vi "SubPanel_DataCollection_Rev11_v10.vi"(0 "DCPowerInformationClusterArray_Input":T7(array[cluster]), 1 "VISAPowerInfoInputArray":T6(array[cluster]), 2 "Run Data SubPanel Input":T5, 3 "RF Block Parameters":T4, 4 "Oscilloscope Info Array":T3(array[cluster]) {"vertical coupling" items=["AC", "DC", "Ground"]}, 6 "New Run?":bool, 7 "error in":errorcluster) -> (20 "DCPowerInformationClusterArray_Output":T7(array[cluster]), 21 "VISAPowerInfoInputOutput":T6(array[cluster]), 22 "Run Data SubPanel Output":T5, 23 "RF Block Parameters Output":T4, 24 "Oscilloscope Info Array Output":T3(array[cluster]) {"vertical coupling" items=["AC", "DC", "Ground"]}, 25 "Reinitialize?":bool, 26 "Data Was Collected?":bool, 27 "error out":errorcluster)   [LabVIEW 2019]
uses:
  Controls/DataBlockControl.ctl
  Controls/QueueDataControl_V3.ctl
  <vilib>/Utility/file.llb/Write Delimited Spreadsheet (string).vi
  Controls/RFBlockControl.ctl
  <instrlib>/niScope/Controls/niScope vertical coupling.ctl
panel:
  out "Current Measurements Live Total":T1(graph)
  out "Voltage Measurements Live Total":T1(graph)
  out "Voltage Measurements Live":T1(graph)
  out "Current Measurements Live":T1(graph)
  out "DCPowerInfoArray":string[][](array[string])
  out "Array":string[][][](array[string])
  out "Current Measurements":cluster{dbl[], dbl[]}[](graph)
  out "Voltage Measurements":cluster{dbl[], dbl[]}[](graph)
  out "Exiting":bool
  out "Full Run Information":string
  out "Ready For Next Run?":bool
  in  "Next Run":bool
  out "Recording Data":bool
  out "Current 2":waveform(dbl)[](graph)
  out "Voltage 2":waveform(dbl)[](graph)
  in  "Record Data Toggle":bool
  out "error of collection":errorcluster
  in  "force exit SubVI":bool
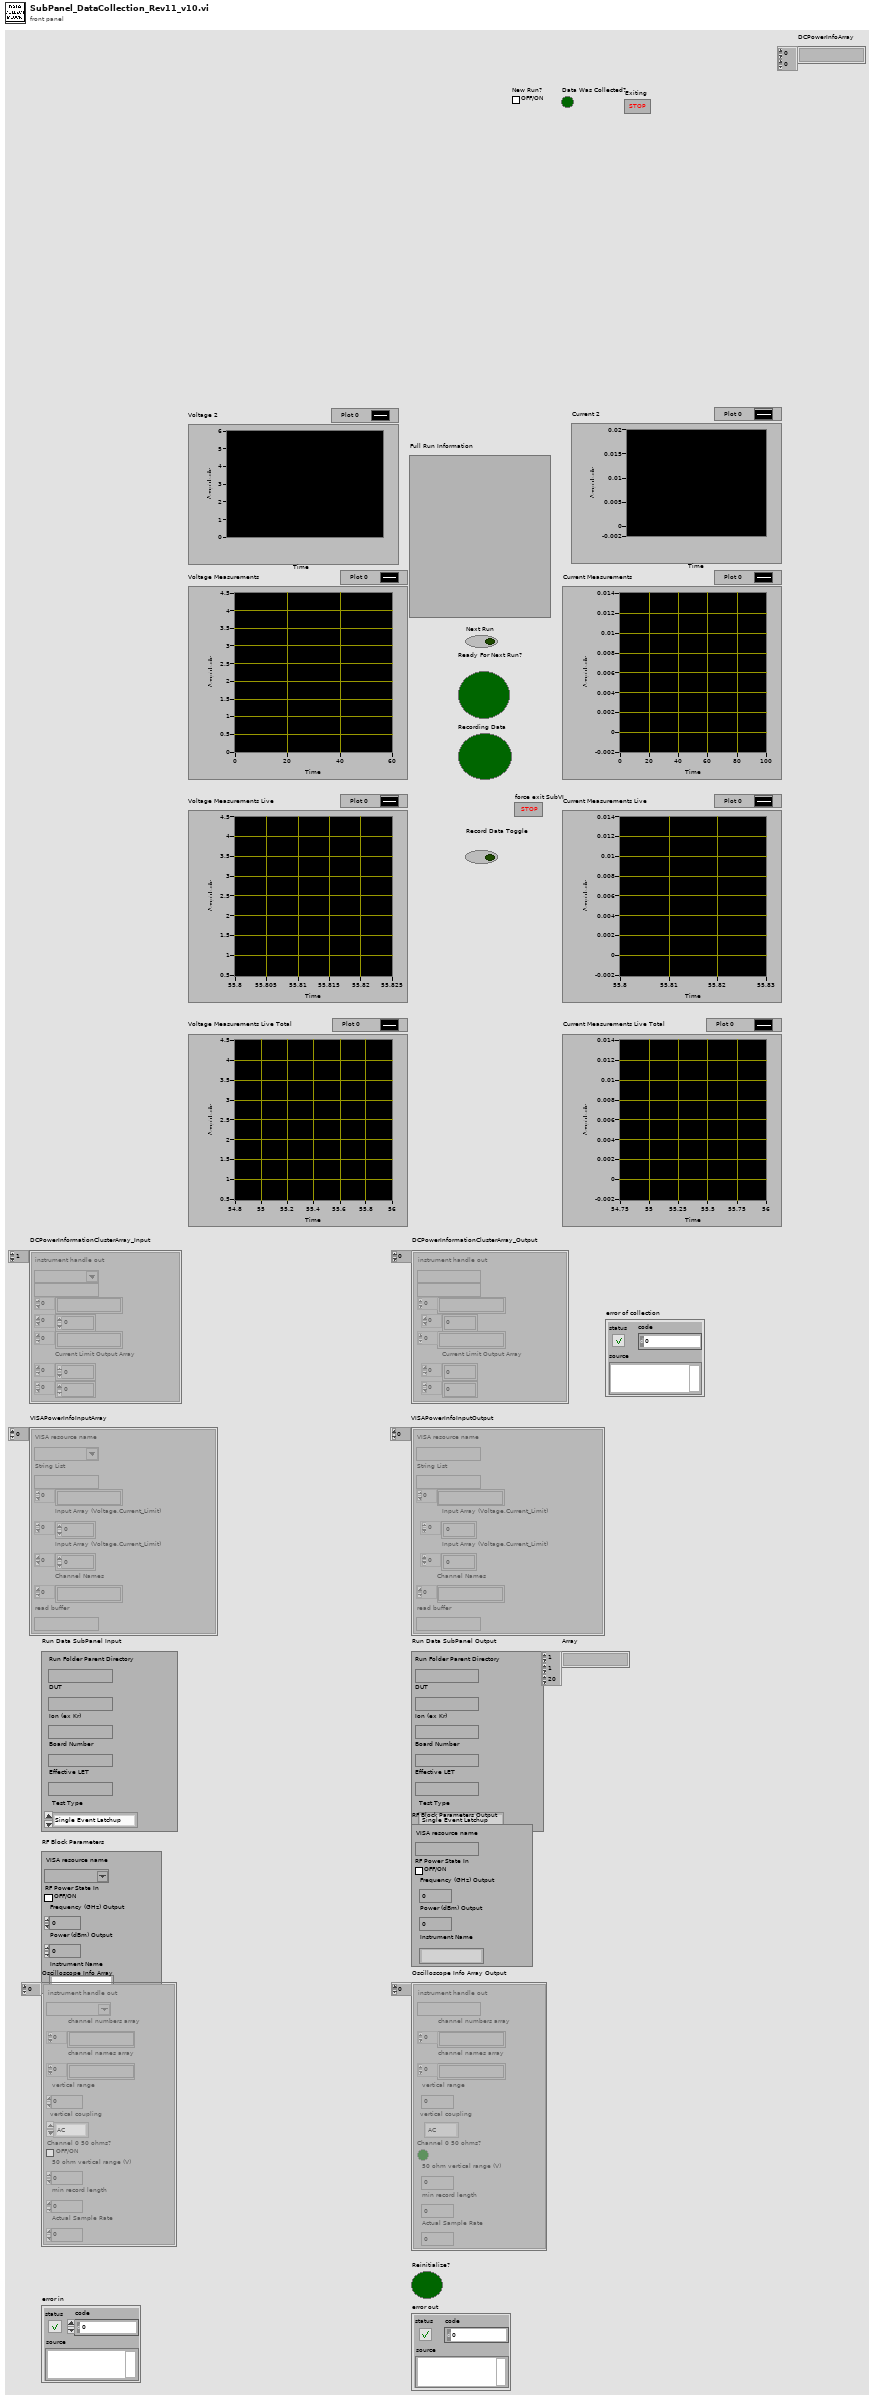
[diagram p1: front panel]
types:
  T1 = cluster{"Array of fetched data":dbl[], "Array of fetched data":dbl[]}[]
  T2 = typedef "niScope vertical coupling.ctl" = i32
  T3 = cluster{"instrument handle out":refnum<k15>, "channel numbers array":string[], "channel names array":string[], "vertical range":dbl, "vertical coupling":T2, "Channel 0 50 ohms?":bool, "50 ohm vertical range (V)":dbl, "min record length":i32, "Actual Sample Rate":dbl}[]
  T4 = typedef "RFBlockControl.ctl" = cluster{"VISA resource name":refnum<visa-resource-name>, "RF Power State In":bool, "Frequency (GHz) Output":dbl, "Power (dBm) Output":dbl, "Instrument Name":string}
  T5 = typedef "DataBlockControl.ctl" = cluster{"Run Folder Parent Directory":path, "DUT":string, "Ion (ex Kr)":string, "Board Number":string, "Effective LET":string, "Test Type":enum16{"Single Event Latchup", "Single Event Transient", "Single Event Upset"}}
  T6 = cluster{"VISA resource name":refnum<visa-resource-name>, "String List":string, string[], "Input Array (Voltage,Current_Limit)":dbl[], "Input Array (Voltage,Current_Limit)":dbl[], "Channel Names":string[], "read buffer":string}[]
  T7 = cluster{"instrument handle out":refnum<k15>, string, string[], dbl[], string[], "Current Limit Output Array":dbl[], dbl[]}[]
  T8 = typedef "QueueDataControl_V3.ctl" = cluster{"Array of fetched data":dbl[][][], "Channel Names Array":string[], "Voltage Waveform Array":waveform(dbl)[], "Current Waveform Array":waveform(dbl)[], "Resetting Time":timestamp}
  T9 = cluster{"IVI Refnum out":refnum<k15>, string, "voltage level channel 23":dbl, "Channel Name 23":string, "Current Limit":dbl, "Measure Record dt":dbl, string}[]
  T10 = cluster{"created path":path, "DCPowerInformation_byChannel":cluster{"IVI Refnum out":refnum<k15>, string, "voltage level channel 23":dbl, "Channel Name 23":string, "Current Limit":dbl, "Measure Record dt":dbl, string}[], string[]}
  T11 = cluster{"Array of fetched data":dbl[][], string, i32[]}
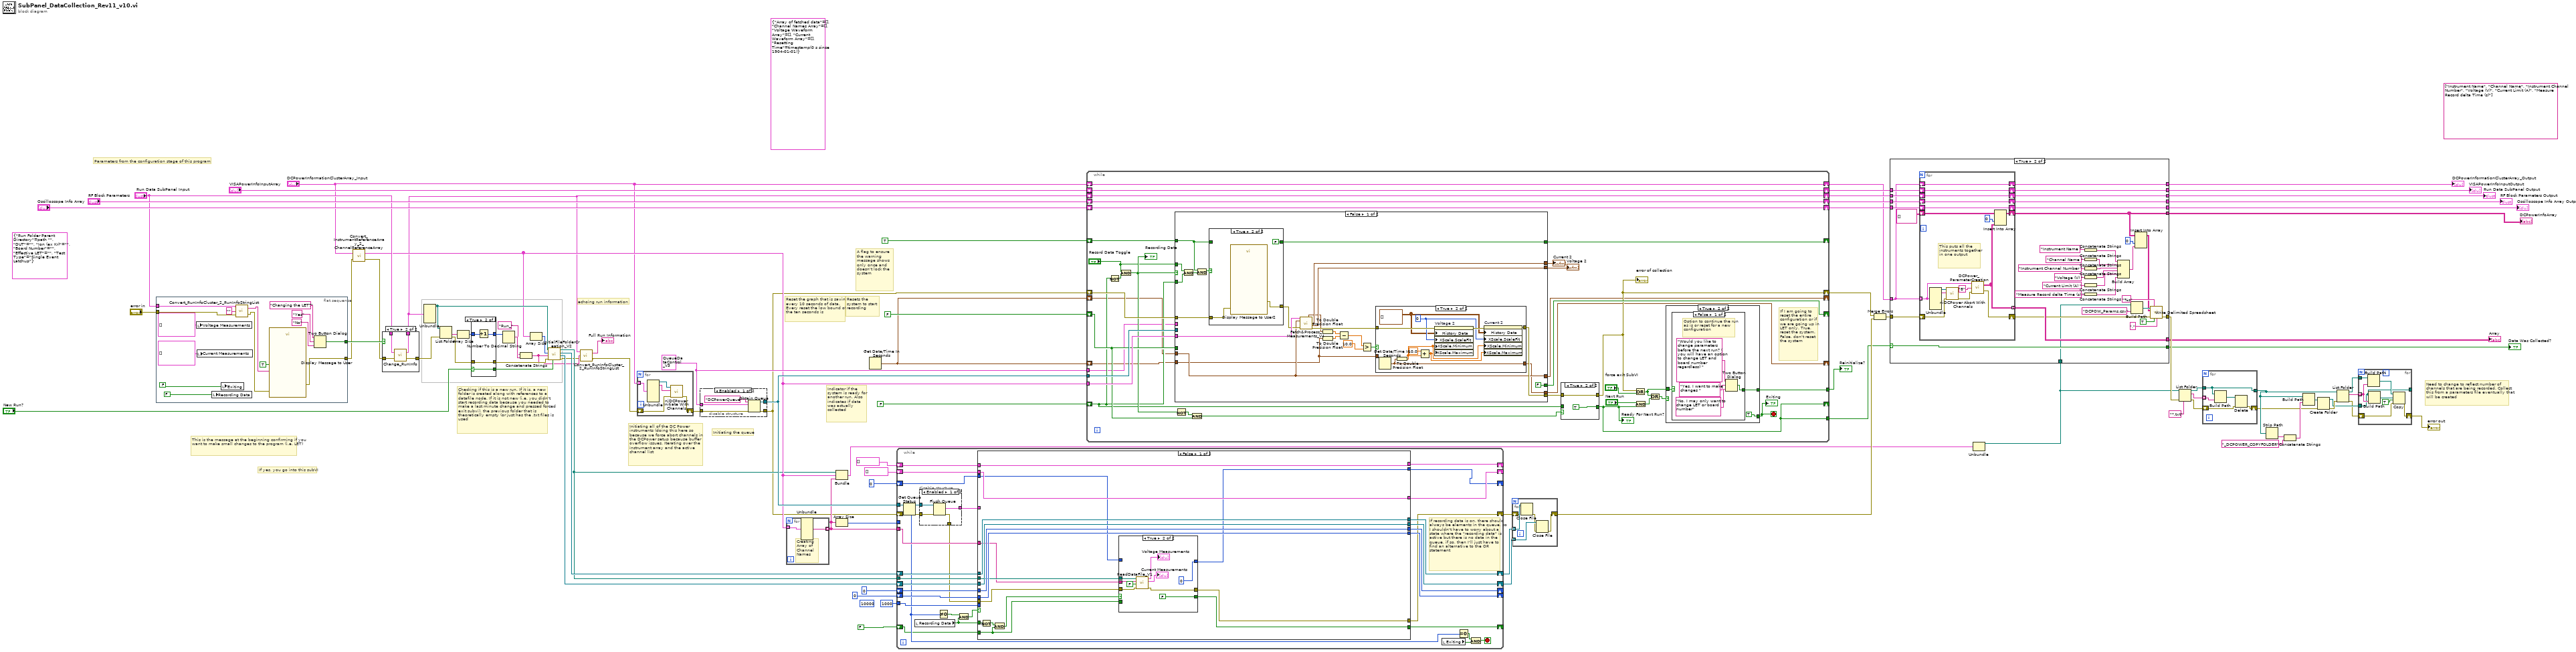
[diagram p0: block diagram]
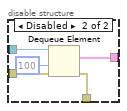
[diagram p2: hidden frame]
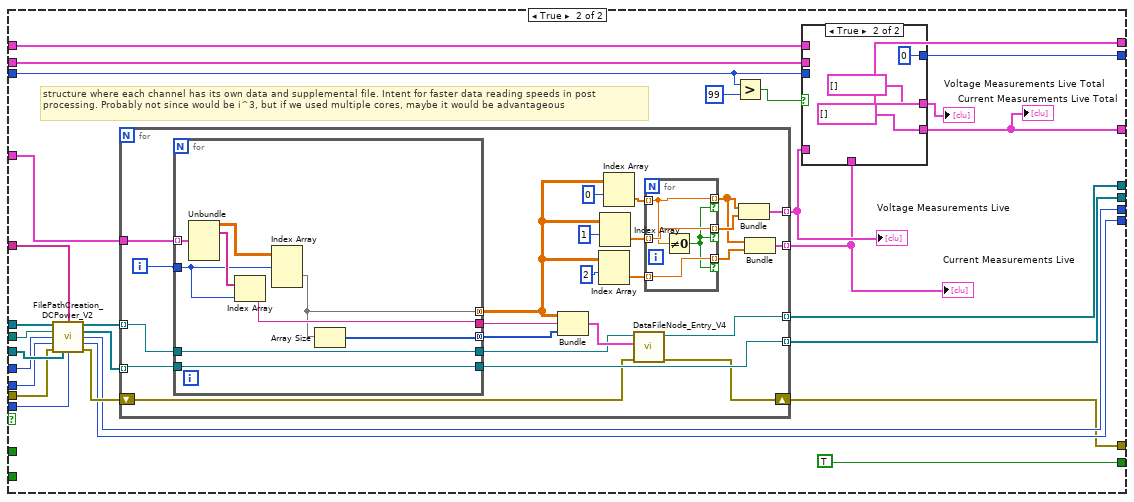
[diagram p4: hidden frame]
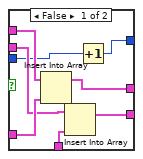
[diagram p5: hidden frame]
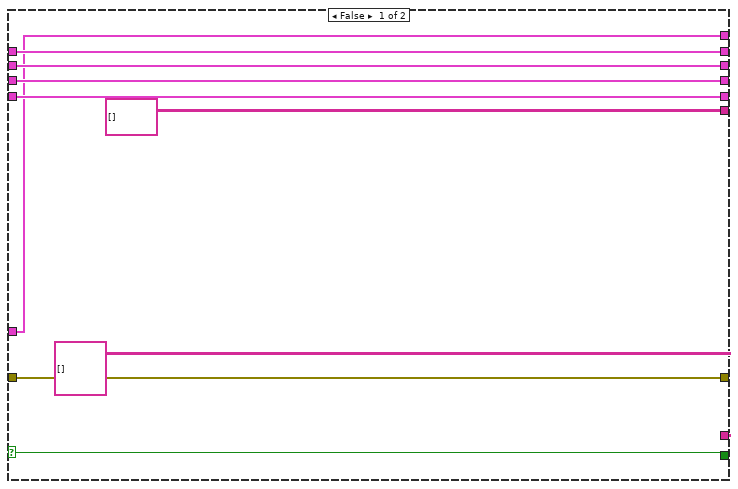
[diagram p6: hidden frame]
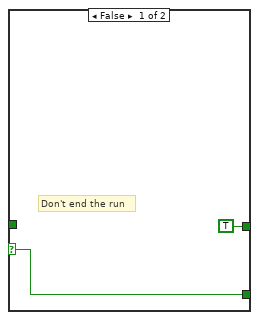
[diagram p10: hidden frame]
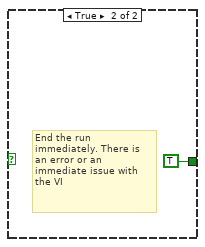
[diagram p11: hidden frame]
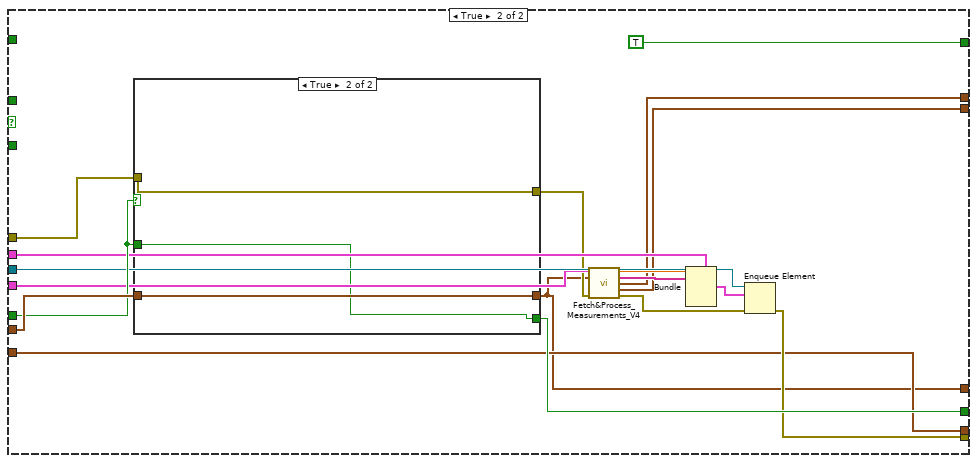
[diagram p15: hidden frame]
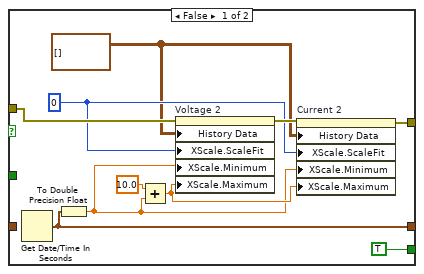
[diagram p16: hidden frame]
diagram:
  (unwired) string[] ["Instrument Name", "Channel Name", "Instrument Channel Number", "Voltage (V)", "Current Limit (A)", "Measure Record delta Time (s)"] ("new element/subarray")
  w57 = T8 {"Array of fetched data"=[], "Channel Names Array"=[], "Voltage Waveform Array"=[], "Current Waveform Array"=[], "Resetting Time"=timestamp(0 s since 1904-01-01)} ("DCPower Queue Data Double Array Format")
  (unwired) T8 {"Array of fetched data"=[], "Channel Names Array"=[], "Voltage Waveform Array"=[], "Current Waveform Array"=[], "Resetting Time"=timestamp(0 s since 1904-01-01)} ("DCPower Double Array Queue")
  (unwired) 10000 ("binary file indexor in")
  (unwired) T5 {"Run Folder Parent Directory"=path "", "DUT"="", "Ion (ex Kr)"="", "Board Number"="", "Effective LET"="", "Test Type"=enum."Single Event Latchup"} ("Run Data Configuration")
  # "Initiating the queue"
  # "echoing run information"
  # "Checking if this is a new run. If it is, a new folder is created along with references to a datafile node. If it is not new (i.e. you didn't start recording data because you needed to make a last minute change and pressed forced exit subvi), the previous folder that is theoretically empty (or just has the .txt files is used"
  # "If yes, you go into this subVI"
  # "This is the message at the beginning confirming if you want to make small changes to the program (i.e. LET)"
  # "Parameters from the configuration stage of this program"
  # "Reset the graph that is saving every 10 seconds of data. Every reset the low bound of the ten seconds is"
  # "Need to change to reflect number of channels that are being recorded. Collect this from a parameters file eventually that will be created"
  # "Indicator if the system is ready for another run. Also indicates if data was actually collected"
  # "Resets the system to start recording"
  # "A flag to ensure the warning message shows only once and doesn't lock the system"
  # "Initiating all of the DC Power instruments (doing this here so because we force abort channels in the DCPower setup because buffer overflow issues. Iterating over the instrument array and the active channel list"
  n1 = flat-sequence {
    tunnel: [w98] -> w73
    tunnel: "error in" -> [w90]
    tunnel: [w102] -> w78
    tunnel: "Run Data SubPanel Input" -> [w89]
    frame #0 {
      n2 = local write "Voltage Measurements"(cluster{dbl[], dbl[]}[] [] ("Voltage Measurements")) -> ()
      n3 = local write "Current Measurements"(cluster{dbl[], dbl[]}[] [] ("Current Measurements")) -> ()
      n4 = local write "Recording Data"(FALSE ("Recording Data")) -> ()
      n5 = local write "Exiting"(FALSE ("Forced Exit")) -> ()
      n6 = call "Convert_RunInfoCluster_2_RunInfoStringList.vi"("error in"=w90, "Run Number"="", "Run Data SubPanel Input"=w89) -> ("error output"=w91:errorcluster, "Run Data Output"=w92:string)
      n7 = call "Display Message to User"("error in (no error)"=w91, "Enable"=TRUE, "Message"=w92) -> ("error out"=w98:errorcluster)  [unwired: 7 in, 1 out]
      n8 = Two Button Dialog(message="Changing the LET?", 1:"No" ("F button name (\"Cancel\")"), 2:"Yes" ("T button name (\"OK\")")) -> (T button?=w102:bool)
    }
  }
  n9 = call "Convert_InstrumentReferenceArray_2_ChannelReferenceArray.vi"("error in (no error)"=w73, "DCPowerInformationClusterArray_Input"="DCPowerInformationClusterArray_Input") -> ("error out"=w72:errorcluster, "DCPowerInformation_byChannel"=w30:T9)
  n10 = case shown="True" w78 {
    tunnel: "Run Data SubPanel Input" -> [w104 w108]
    tunnel: [w104 w107] -> w7
    tunnel: [w103 w106] -> w74
    tunnel: w72 -> [w103 w105]
    frame False {
    }
    frame True {
      n11 = call "Change_RunInfo.vi"("error in (no error)"=w105, "Run Data SubPanel in"=w108) -> ("error out"=w106:errorcluster, "Run Data SubPanel out"=w107:T5)
    }
  }
  n12 = Unbundle(w7) -> ("Run Folder Parent Directory"=w75:path)  [unwired: 5 out]
  n13 = List Folder(path=w75, error in=w74) -> (folder names=w76:string[], error out=w60:errorcluster)  [unwired: 2 in, 2 out]
  n14 = Array Size(array=w76) -> (size(s)=w63:i32)
  n15 = case shown="True" "New Run?" {
    selector: "New Run?" -> [w110 w113]
    tunnel: [w111 w115] -> w64
    tunnel: w63 -> [w111 w114]
    tunnel: [w110 w113] -> w62
    tunnel: [w109 w112] -> w61
    tunnel: w60 -> [w109 w112]
    frame False {
    }
    frame True {
      n16 = Increment(x=w114) -> (x+1=w115:i32)
    }
  }
  n17 = Number To Decimal String(number=w64) -> (decimal integer string=w67:string)  [unwired: 1 in]
  n18 = Concatenate Strings("Run_", w67) -> (w6:string)
  n19 = Array Size(array=w30) -> (size(s)=w59:i32)
  n20 = call "InitialFileFolderCreation_V2.vi"("New Run?"=w62, "error in (no error)"=w61, "Run Number"=w6, "DCPowerArrayClusterSize"=w59, "base path"=w75) -> ("error out"=w5:errorcluster, "SupplementalDataFileReferenceObjectArray"=w70:refnum<file>[], "DataFileReferenceObjectArray"=w71:refnum<file>[], "created path"=w14:path)  [unwired: 3 in]
  n21 = call "Convert_RunInfoCluster_2_RunInfoStringList.vi"("error in"=w5, "Run Number"=w6, "Run Data SubPanel Input"=w7) -> ("error output"=w4:errorcluster, "Run Data Output"=→"Full Run Information":string)
  n22 = for {
    shift-right: [w116] -> w12
    shift-left: w4 -> [w118]
    tunnel: "DCPowerInformationClusterArray_Input" -> [w120] mode=indexing
    n23 = Unbundle(w120) -> ("instrument handle out"=w117:refnum<k15>, w119:string)  [unwired: 5 out]
    n24 = call <instrlib>:"niDCPower Initiate With Channels.vi"("error in (no error)"=w118, "channel name"=w119, "instrument handle"=w117) -> ("error out"=w116:errorcluster)  [unwired: 7 in, 1 out]
  }
  n25 = disable-structure shown="Enabled" {
    disable-tunnel: w12 -> [w124 w126]
    disable-tunnel: [w123 w126] -> w9
    disable-tunnel: [w122 _] -> w83
    disable-tunnel: w57 -> [w121 _]
    frame Enabled {
      n26 = Obtain Queue(name (unnamed)="DCPowerQueue", element data type=w121, error in (no error)=w124) -> (queue out=w122:refnum<queue>, error out=w123:errorcluster)  [unwired: 2 in, 1 out]
    }
    frame Disabled {
    }
  }
  n27 = for {
    tunnel: w30 -> [w128] mode=indexing
    tunnel: [w127] -> w31 mode=indexing
    # "Creating Array of Channel Names"
    n28 = Unbundle(w128) -> ("Channel Name 23"=w127:string)  [unwired: 6 out]
  }
  n29 = Bundle("created path"=w14, "DCPowerInformation_byChannel"=w30, w31) -> (w29:T10)  [unwired: 1 in]
  n30 = Array Size(array=w31) -> (size(s)=w52:i32)
  n31 = Get Date/Time In Seconds() -> (seconds since 1Jan1904=w10:timestamp)
  n32 = while {
    tunnel: w83 -> [w161]
    shift-right: [w148] -> w54
    shift-left: w9 -> [w160]
    tunnel: w14 -> [w157]
    shift-right: [w150] -> w56
    shift-left: w71 -> [w158]
    shift-right: [w149] -> w55
    shift-left: w70 -> [w156]
    shift-right: [w152] -> _
    shift-left: 0 ("binary file indexor in") -> [w155]
    shift-right: [w151] -> _
    shift-left: 0 ("binary file indexor in") -> [w154]
    tunnel: 1000 ("binary file indexor in") -> [w153]
    tunnel: w31 -> [w159]
    tunnel: w52 -> [_]
    shift-right: [w137] -> _
    shift-left: FALSE -> [w136]
    shift-right: [w133] -> _
    shift-left: T1 [] ("array") -> [w134]
    shift-right: [w131] -> _
    shift-left: T1 [] ("array") -> [w132]
    shift-right: [w129] -> _
    shift-left: 0 -> [w130]
    stop <- w145 stop-if-true
    # "If recording data is on, there should always be elements in the queue, so I shouldn't have to worry about a state where the \"recording data\" is active but there is no data in the queue, if so, then I'll just have to find an alternative to the OR statement"
    n33 = Get Queue Status(queue=w161, error in (no error)=w160) -> (queue out=w142:refnum<queue>, error out=w143:errorcluster, # elements in queue=w138:i32)  [unwired: 1 in, 5 out]
    n34 = local read "Recording Data"() -> (w135:bool)
    n35 = disable-structure shown="Enabled" {
      disable-tunnel: [w165 w167] -> w144
      disable-tunnel: w143 -> [w164 w169]
      disable-tunnel: w142 -> [w163 w170]
      disable-tunnel: [w162 w166] -> w141
      frame Enabled {
        n36 = Flush Queue(queue=w163, error in (no error)=w164) -> (remaining elements=w162:T8[], error out=w165:errorcluster)  [unwired: 1 out]
      }
      frame Disabled {
        n37 = Dequeue Element(queue=w170, timeout in ms (-1)=100, error in (no error)=w169) -> (element=w166:T8, error out=w167:errorcluster)  [unwired: 2 out]
      }
    }
    n38 = Not Equal To 0?(x=w138) -> (x != 0?=w140:bool)
    n39 = And(x=w140, y=w135) -> (x .and. y?=w139:bool)
    n40 = case shown="False" w139 {
      tunnel: w141 -> [_ w227]
      tunnel: w144 -> [w178 w221]
      tunnel: w159 -> [w179 w213]
      tunnel: w158 -> [w186 w226]
      tunnel: w157 -> [w180 w225]
      tunnel: w156 -> [w187 w224]
      tunnel: w155 -> [w185 w223]
      tunnel: w154 -> [w184 w212]
      tunnel: w153 -> [_ w211]
      tunnel: [w185 w220] -> w152
      tunnel: [w184 w219] -> w151
      tunnel: [w186 w216] -> w150
      tunnel: [w187 w215] -> w149
      tunnel: [w177 w214] -> w148
      tunnel: [w176 TRUE] -> w137
      tunnel: w136 -> [w175 _]
      tunnel: w135 -> [w183 _]
      tunnel: w134 -> [w174 w207]
      tunnel: [w174 w206] -> w133
      tunnel: w132 -> [w173 w205]
      tunnel: [w173 w204] -> w131
      tunnel: w130 -> [w172 w201]
      tunnel: [w171 w200] -> w129
      frame False {
        n41 = Not(x=w183) -> (.not. x?=w182:bool)
        n42 = And(x=w182, y=w175) -> (x .and. y?=w181:bool)
        n43 = case shown="True" w181 {
          tunnel: w180 -> [_ w199]
          tunnel: w179 -> [_ w198]
          tunnel: w178 -> [w190 w196]
          tunnel: [w190 w195] -> w177
          tunnel: [w189 FALSE] -> w176
          tunnel: w175 -> [w189 _]
          tunnel: w172 -> [w188 _]
          tunnel: [w188 0] -> w171
          frame False {
          }
          frame True {
            n44 = call "ReadDataFile_V1.vi"("error in (no error)"=w196, "Create CSV files?"=FALSE, "Channel Names Array"=w198, "DataFolder Path"=w199) -> ("error out"=w195:errorcluster, "Current Measurements"=→"Current Measurements":cluster{dbl[], dbl[]}[], "Voltage Measurements"=→"Voltage Measurements":cluster{dbl[], dbl[]}[])  [unwired: 5 in]
          }
        }
      }
      frame True {
        # "structure where each channel has its own data and supplemental file. Intent for faster data reading speeds in post processing. Probably not since would be i^3, but if we used multiple cores, maybe it would be advantageous"
        n45 = call "FilePathCreation_DCPower_V2.vi"("binary file input reference array 1"=w226, "Channel Name Input array"=w213, "data output directory folder"=w225, "binary file indexor in"=w223, "Reset counter in"=w212, "error in (no error)"=w221, "binary file input reference array 2"=w224, "reset threshold"=w211) -> ("binary file output reference array"=w218:refnum<file>[], "binary file output reference array 2"=w217:refnum<file>[], "binary file indexor out"=w220:i32, "reset counter out"=w219:i32, "error out"=w222:errorcluster)  [unwired: 3 in]
        n46 = for {
          shift-right: [w252] -> w214
          shift-left: w222 -> [w253]
          tunnel: w227 -> [w262]
          tunnel: w217 -> [w259] mode=indexing
          tunnel: w218 -> [w258] mode=indexing
          tunnel: [w257] -> w215 mode=indexing
          tunnel: [w251] -> w216 mode=indexing
          tunnel: [w246] -> w209 mode=indexing
          tunnel: [w245] -> w208 mode=indexing
          i -> [w256]
          n47 = for {
            tunnel: w262 -> [w275] mode=indexing
            tunnel: w256 -> [w272]
            tunnel: [w267] -> w247 mode=concatenating
            tunnel: [w271] -> w261
            tunnel: w259 -> [w270]
            tunnel: w258 -> [w268]
            tunnel: [w268] -> w254
            tunnel: [w270] -> w257
            tunnel: [w269] -> w260 mode=concatenating
            n48 = Unbundle(w275) -> ("Array of fetched data"=w274:dbl[][][], "Channel Names Array"=w273:string[])  [unwired: 3 out]
            n49 = Index Array(array=w273, index=w272) -> (element=w271:string)
            n50 = Index Array(array=w274, index (dim 0)=w272) -> (element=w267:dbl[][])  [unwired: 2 in]
            n51 = Array Size(array=w267) -> (size(s)=w269:i32[])
          }
          n52 = Bundle("Array of fetched data"=w247, w261, w260) -> (w255:T11)  [unwired: 1 in]
          n53 = Index Array(array=w247, index (row)=2) -> (element=w240:dbl[])  [unwired: 1 in]
          n54 = Index Array(array=w247, index (row)=1) -> (element=w242:dbl[])  [unwired: 1 in]
          n55 = Index Array(array=w247, index (row)=0) -> (element=w244:dbl[])  [unwired: 1 in]
          n56 = call "DataFileNode_Entry_V4.vi"("error in (no error)"=w253, "Queued Elements"=w255, "Byte Stream File in"=w254) -> ("error out"=w252:errorcluster, "Byte Stream File out"=w251:refnum<file>)  [unwired: 7 in]
          n57 = for {
            tunnel: [w264] -> w239 mode=indexing if=w263
            tunnel: w244 -> [w264] mode=indexing
            tunnel: [w266] -> w243 mode=indexing if=w263
            tunnel: w242 -> [w266] mode=indexing
            tunnel: [w265] -> w241 mode=indexing if=w263
            tunnel: w240 -> [w265] mode=indexing
            n58 = Not Equal To 0?(x=w264) -> (x != 0?=w263:bool)
          }
          n59 = Bundle(w239, w243) -> (w246:cluster{dbl[], dbl[]})  [unwired: 1 in]
          n60 = Bundle(w239, w241) -> (w245:cluster{dbl[], dbl[]})  [unwired: 1 in]
        }
        "Current Measurements Live" <- w208
        "Voltage Measurements Live" <- w209
        n61 = Greater?(x=w201, y=99) -> (0:w203:bool)
        n62 = case shown="True" w203 {
          tunnel: w209 -> [w235 _]
          tunnel: w208 -> [w234 _]
          tunnel: w207 -> [w233 _]
          tunnel: [w232 T1 [] ("array")] -> w206
          tunnel: w205 -> [w231 _]
          tunnel: [w230 T1 [] ("array")] -> w204
          tunnel: w201 -> [w229 _]
          tunnel: [w228 0] -> w200
          frame False {
            n63 = Insert Into Array(array=w233, new element=w235) -> (w232:T1)  [unwired: 1 in]
            n64 = Insert Into Array(array=w231, new element=w234) -> (w230:T1)  [unwired: 1 in]
            n65 = Increment(x=w229) -> (x+1=w228:i32)
          }
          frame True {
          }
        }
        "Voltage Measurements Live Total" <- w206
        "Current Measurements Live Total" <- w204
      }
    }
    n66 = local read "Exiting"() -> (w147:bool)
    n67 = Equal To 0?(x=w138) -> (x = 0?=w146:bool)
    n68 = And(x=w146, y=w147) -> (x .and. y?=w145:bool)
  }
  n69 = while {
    shift-right: [w306] -> w19
    shift-left: "DCPowerInformationClusterArray_Input" -> [w306]
    shift-right: [w310] -> w21
    shift-left: "VISAPowerInfoInputArray" -> [w310]
    shift-right: [w309] -> w23
    shift-left: w7 -> [w309]
    shift-right: [w308] -> w25
    shift-left: "RF Block Parameters" -> [w308]
    shift-right: [w307] -> w27
    shift-left: "Oscilloscope Info Array" -> [w307]
    shift-right: [w291] -> w58
    shift-left: w9 -> [w304]
    tunnel: w30 -> [w305]
    shift-right: [w301] -> _
    shift-left: FALSE -> [w298]
    tunnel: w83 -> [w300]
    shift-right: [w280] -> _
    shift-left: FALSE -> [w285]
    tunnel: [w289] -> w82
    shift-right: [w283] -> _
    shift-left: TRUE ("x .and. y?") -> [w284]
    shift-right: [w281] -> _
    shift-left: w10 -> [w282]
    tunnel: [w280] -> w18
    tunnel: w57 -> [w278]
    shift-right: [w276] -> _
    shift-left: w10 -> [w277]
    stop <- w279 stop-if-true
    # "If I am going to reset the entire configuration or if we are going up in LET only. True, reset the system. False, don't reset the system"
    n70 = Not(x=w285) -> (.not. x?=w287:bool)
    n71 = And(x="Record Data Toggle", y=w287) -> (x .and. y?=w288:bool)
    "Recording Data" <- w288
    n72 = case shown="False" w288 {
      tunnel: w305 -> [w347 w371]
      tunnel: w304 -> [w344 w379]
      tunnel: [w333 w366] -> w303
      tunnel: [w334 w365] -> w302
      tunnel: w298 -> [_ w377]
      tunnel: [FALSE w378] -> w301
      tunnel: w300 -> [_ w376]
      tunnel: [w345 w375] -> w296
      tunnel: "Record Data Toggle" -> [w341 _]
      tunnel: w285 -> [w342 _]
      tunnel: w284 -> [w337 _]
      tunnel: [w338 TRUE] -> w283
      tunnel: w282 -> [w336 w380]
      tunnel: [w336 w369] -> w281
      tunnel: w278 -> [_ w374]
      tunnel: w277 -> [w332 w372]
      tunnel: [w335 w372] -> w276
      frame False {
        n73 = And(x=w341, y=w342) -> (x .and. y?=w340:bool)
        n74 = And(x=w337, y=w340) -> (x .and. y?=w339:bool)
        n75 = case shown="True" w339 {
          tunnel: [w360 w362] -> w343
          tunnel: w344 -> [w360 w363]
          tunnel: [w359 FALSE] -> w338
          tunnel: w337 -> [w359 _]
          frame False {
          }
          frame True {
            n76 = call "Display Message to User2"("error in (no error)"=w363) -> ("error out"=w362:errorcluster)  [unwired: 9 in, 1 out]
          }
        }
        n77 = call "Fetch&Process_Measurements_V4.vi"("DCPowerInformation_byChannel"=w347, "Initial Time"=w336, "error in (no error)"=w343) -> ("Latest Time"=w330:timestamp, "Current Waveform Array"=w333:waveform(dbl)[], "Voltage Waveform Array"=w334:waveform(dbl)[], "error out"=w331:errorcluster)  [unwired: 6 in, 3 out]
        n78 = To Double Precision Float(number=w330) -> (double precision float=w328:dbl)
        n79 = To Double Precision Float(number=w332) -> (double precision float=w329:dbl)
        n80 = Subtract(x=w328, y=w329) -> (x-y=w327:dbl)
        n81 = Greater?(x=w327, y=10.0) -> (0:w325:bool)
        n82 = case shown="True" w325 {
          tunnel: w331 -> [w348 w358]
          tunnel: [w349 w355] -> w335
          tunnel: w332 -> [w349 _]
          tunnel: [w348 w356] -> w345
          frame False {
          }
          frame True {
            w354 = u8 0 ("X Scale.Scale Fit")
            w353 = waveform(dbl)[][] [] ("History Data")
            n83 = Get Date/Time In Seconds() -> (seconds since 1Jan1904=w355:timestamp)
            n84 = To Double Precision Float(number=w355) -> (double precision float=w351:dbl)
            n85 = Add(x=10.0, y=w351) -> (x+y=w350:dbl)
            n86 = property on="Voltage 2" class="WFChart (strict)"(error in=w358, "History Data"=w353, "XScale.ScaleFit"=w354, "XScale.Minimum"=w351, "XScale.Maximum"=w350) -> (error out=w357:errorcluster)  [unwired: 1 in, 1 out]
            n87 = property on="Current 2" class="WFChart (strict)"(error in=w357, "History Data"=w353, "XScale.ScaleFit"=w354, "XScale.Minimum"=w351, "XScale.Maximum"=w350) -> (error out=w356:errorcluster)  [unwired: 1 in, 1 out]
          }
        }
      }
      frame True {
        n88 = case shown="True" w377 {
          tunnel: [w386 w394] -> w369
          tunnel: w380 -> [_ w394]
          tunnel: w379 -> [w391 w393]
          tunnel: [w389 w393] -> w370
          tunnel: [TRUE w392] -> w378
          tunnel: w377 -> [_ w392]
          frame False {
            w382 = waveform(dbl)[][] [] ("History Data")
            w387 = u8 0 ("X Scale.Scale Fit")
            n89 = Get Date/Time In Seconds() -> (seconds since 1Jan1904=w386:timestamp)
            n90 = To Double Precision Float(number=w386) -> (double precision float=w383:dbl)
            n91 = Add(x=10.0 ("y"), y=w383) -> (x+y=w385:dbl)
            n92 = property on="Voltage 2" class="WFChart (strict)"(error in=w391, "History Data"=w382, "XScale.ScaleFit"=w387, "XScale.Minimum"=w383, "XScale.Maximum"=w385) -> (error out=w390:errorcluster)  [unwired: 1 in, 1 out]
            n93 = property on="Current 2" class="WFChart (strict)"(error in=w390, "History Data"=w382, "XScale.ScaleFit"=w387, "XScale.Minimum"=w383, "XScale.Maximum"=w385) -> (error out=w389:errorcluster)  [unwired: 1 in, 1 out]
          }
          frame True {
          }
        }
        n94 = call "Fetch&Process_Measurements_V4.vi"("DCPowerInformation_byChannel"=w371, "Initial Time"=w369, "error in (no error)"=w370) -> ("Data As dbl Array"=w368:dbl[][][], "Channel Number Array"=w367:string[], "Current Waveform Array"=w366:waveform(dbl)[], "Voltage Waveform Array"=w365:waveform(dbl)[], "error out"=w364:errorcluster)  [unwired: 6 in, 2 out]
        n95 = Bundle(cluster=w374, "Array of fetched data"=w368, "Channel Names Array"=w367) -> (w373:T8)  [unwired: 3 in]
        n96 = Enqueue Element(queue=w376, element=w373, error in (no error)=w364) -> (error out=w375:errorcluster)  [unwired: 1 in, 2 out]
      }
    }
    "Voltage 2" <- w302
    "Current 2" <- w303
    n97 = Not(x=w288) -> (.not. x?=w299:bool)
    n98 = And(x=w299, y=w298) -> (x .and. y?=w297:bool)
    n99 = case shown="True" w297 {
      tunnel: w296 -> [w321 w323]
      tunnel: [w322 TRUE] -> w280
      tunnel: w285 -> [w322 _]
      tunnel: [w321 w323] -> w291
      frame False {
      }
      frame True {
      }
    }
    "error of collection" <- w291
    "Ready For Next Run?" <- w280
    n100 = Or(x=w291, y="force exit SubVI") -> (x .or. y?=w293:bool)
    n101 = And(x="Next Run", y=w280) -> (x .and. y?=w295:bool)
    n102 = Or(x=w293, y=w295) -> (x .or. y?=w294:bool)
    n103 = case shown="True" w294 {
      selector: w294 -> [w312 _]
      tunnel: w293 -> [_ w315]
      tunnel: [w312 TRUE] -> w279
      tunnel: [TRUE ("T button?") w313] -> w289
      frame False {
        # "Don't end the run"
      }
      frame True {
        n104 = case shown="False" w315 {
          tunnel: [w316 TRUE] -> w313
          frame False {
            # "Option to continue the run as is or reset for a new configuration"
            n105 = Two Button Dialog(message="Would you like to change parameters before the next run? ( you will have an option to change LET and board number regardless) ", 1:"No, I may only want to change LET or board number" ("F button name (\"Cancel\")"), 2:"Yes, I want to make changes " ("T button name (\"OK\")")) -> (T button?=w316:bool)
          }
          frame True {
            # "End the run immediately. There is an error or an immediate issue with the VI"
          }
        }
      }
    }
    "Exiting" <- w279
  }
  "Reinitialize?" <- w82
  n106 = for {
    tunnel: w56 -> [w399] mode=indexing
    tunnel: w55 -> [w397] mode=indexing
    shift-right: [w395] -> w53
    shift-left: w54 -> [w398]
    n107 = Close File(refnum=w399, error in=w398) -> (error out=w396:errorcluster)  [unwired: 1 out]
    n108 = Close File(refnum=w397, error in=w396) -> (error out=w395:errorcluster)  [unwired: 1 out]
  }
  n109 = Merge Errors(w58, w53) -> (w33:errorcluster)
  n110 = Unbundle(w29) -> ("created path"=w13:path)  [unwired: 2 out]
  n111 = case shown="True" w18 {
    selector: w18 -> [w403 w435]
    tunnel: w33 -> [w402 w446]
    tunnel: [w402 w429] -> w32
    tunnel: [w408 w445] -> w28
    tunnel: w27 -> [w408 w444]
    tunnel: [w407 w443] -> w26
    tunnel: w25 -> [w407 w442]
    tunnel: [w406 w441] -> w24
    tunnel: w23 -> [w406 w440]
    tunnel: [w405 w439] -> w22
    tunnel: w21 -> [w405 w438]
    tunnel: [w404 w437] -> w20
    tunnel: w19 -> [w404 w436]
    tunnel: [w403 w435] -> w17
    tunnel: [string[][][] [] w434] -> w16
    tunnel: [string[][] [] ("DCPowerInfoArray") w424] -> w15
    tunnel: w13 -> [_ w427]
    frame False {
    }
    frame True {
      n112 = for {
        shift-right: [w448] -> w430
        shift-left: w446 -> [w460]
        tunnel: w436 -> [w451] mode=indexing
        shift-right: [w459] -> w445
        shift-left: w444 -> [w459]
        shift-right: [w458] -> w443
        shift-left: w442 -> [w458]
        shift-right: [w457] -> w441
        shift-left: w440 -> [w457]
        shift-right: [w456] -> w439
        shift-left: w438 -> [w456]
        shift-right: [w455] -> w437
        shift-left: w436 -> [w455]
        tunnel: [w447] -> w434 mode=indexing
        shift-right: [w453] -> w424
        shift-left: string[][] [] ("DCPowerInfoArray") -> [w454]
        # "This puts all the instruments together in one output"
        n113 = Unbundle(w451) -> ("instrument handle out"=w462:refnum<k15>, w461:string)  [unwired: 5 out]
        n114 = call <instrlib>:"niDCPower Abort With Channels.vi"("error in (no error)"=w460, "channel name"=w461, "instrument handle"=w462) -> ("error out"=w449:errorcluster)  [unwired: 7 in, 1 out]
        n115 = call "DCPower_ParameterCreation.vi"("error in"=w449, "Precision"="8", "DCPowerInformationByInstrument"=w451) -> ("error out"=w448:errorcluster, "DCPowerInfoArray"=w447:string[][])
        n116 = Insert Into Array(array=w454, index (col)=0 ("disabled index (col)"), new element=w447) -> (w453:string[][])  [unwired: 1 in]
      }
      n117 = Concatenate Strings("Channel Name " ("string")) -> (w419:string)
      n118 = Concatenate Strings("Voltage (V) " ("string")) -> (w421:string)
      n119 = Concatenate Strings("Measure Record delta Time (s) " ("string")) -> (w423:string)
      n120 = Concatenate Strings("Instrument Name " ("string")) -> (w418:string)
      n121 = Concatenate Strings("Instrument Channel Number " ("string")) -> (w420:string)
      n122 = Concatenate Strings("Current Limit (A) " ("string")) -> (w422:string)
      n123 = Build Array(w418, w419, w420, w421, w422, w423) -> (w411:string[])
      n124 = Build Path(base path=w427, name or relative path="DCPOW_Params.csv") -> (appended path=w428:path)
      n125 = Insert Into Array(array=w424, index (col)=0 ("disabled index (col)"), new element=w411) -> (w410:string[][])  [unwired: 1 in]
      n126 = call-poly <vilib>:"Write Delimited Spreadsheet.vi"("file path (dialog if empty)"=w428, "format (%s)"="%s" ("format (%.3f)"), "2D data"=w410, "error in (no error)"=w430, "transpose? (no:F)"=TRUE, "delimiter (\\t)"="," ("delimiter (\\t)")) -> ("error out"=w429:errorcluster)  [unwired: 8 in, 1 out]
    }
  }
  "DCPowerInformationClusterArray_Output" <- w20
  "VISAPowerInfoInputOutput" <- w22
  "Run Data SubPanel Output" <- w24
  "RF Block Parameters Output" <- w26
  "Oscilloscope Info Array Output" <- w28
  "Data Was Collected?" <- w17
  "Array" <- w16
  "DCPowerInfoArray" <- w15
  n127 = List Folder(path=w13, pattern="*.txt", error in=w32) -> (path out=w38:path, filenames=w37:string[], error out=w36:errorcluster)  [unwired: 1 in, 1 out]
  n128 = for {
    tunnel: [w463] -> w39
    tunnel: w38 -> [w463]
    tunnel: w37 -> [w465] mode=indexing
    shift-right: [w466] -> w35
    shift-left: w36 -> [w467]
    n129 = Build Path(base path=w463, name or relative path=w465) -> (appended path=w464:path)
    n130 = Delete(path (use dialog)=w464, error in=w467) -> (error out=w466:errorcluster)  [unwired: 3 in, 2 out]
  }
  n131 = Strip Path(path=w39) -> (name=w43:string)  [unwired: 1 out]
  n132 = Concatenate Strings(w43, "_DCPOWER_COPYFOLDER" ("name or relative path")) -> (w41:string)
  n133 = Build Path(base path=w39, name or relative path=w41) -> (appended path=w50:path)
  n134 = Create Folder(path (use dialog)=w50, error in=w35) -> (created path=w45:path, error out=w48:errorcluster)  [unwired: 1 in, 1 out]
  n135 = List Folder(path=w39, error in=w48) -> (path out=w47:path, filenames=w46:string[], error out=w44:errorcluster)  [unwired: 2 in, 1 out]
  n136 = for {
    tunnel: w47 -> [w473]
    tunnel: w46 -> [w472] mode=indexing
    tunnel: w45 -> [w468]
    shift-right: [w475] -> w49
    shift-left: w44 -> [w469]
    tunnel: [w468] -> _
    n137 = Build Path(base path=w473, name or relative path=w472) -> (appended path=w470:path)
    n138 = Build Path(base path=w468, name or relative path=w472) -> (appended path=w471:path)
    n139 = Copy(8:w469, 9:TRUE ("overwrite (F)"), 10:w471, 11:w470) -> (0:w475:errorcluster)  [unwired: 1 in, 2 out]
  }
  "error out" <- w49
